vi "DCP SORT.vi"(11 "Clusters in":T1) -> (3 "Array":string[][](array[string]))   [LabVIEW 2015]
uses:
  TypeDefs/DCP and LLDP Cluster.ctl
  TypeDefs/DCP ARRAY.ctl
  TypeDefs/Profinet Ident.ctl
  TypeDefs/LLDP ARRAY.ctl
  TypeDefs/LLDP.ctl
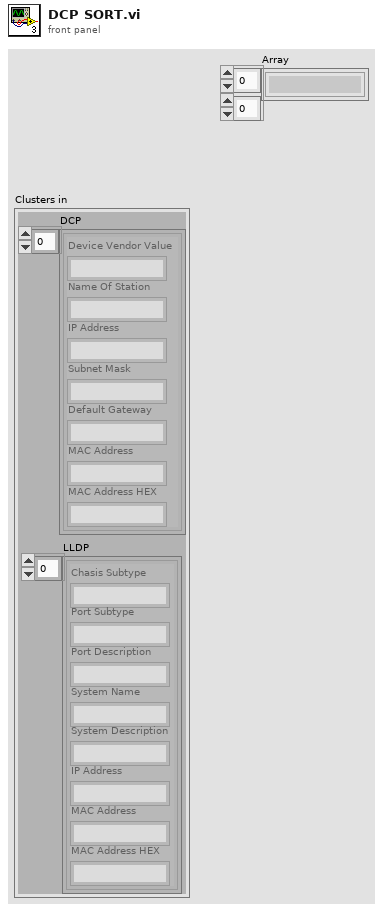
[diagram p1: front panel]
types:
  T1 = typedef "DCP and LLDP Cluster.ctl" = cluster{"DCP":T2, "LLDP":T4}
  T2 = typedef "DCP ARRAY.ctl" = T3[]
  T3 = typedef "Profinet Ident.ctl" = cluster{"Device Vendor Value":string, "Name Of Station":string, "IP Address":string, "Subnet Mask":string, "Default Gateway":string, "MAC Address":string, "MAC Address HEX":string}
  T4 = typedef "LLDP ARRAY.ctl" = T5[]
  T5 = typedef "LLDP.ctl" = cluster{"Chasis Subtype":string, "Port Subtype":string, "Port Description":string, "System Name":string, "System Description":string, "IP Address":string, "MAC Address":string, "MAC Address HEX":string}
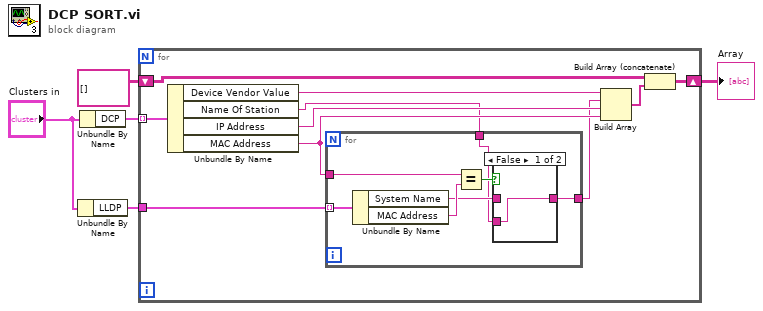
[diagram p0: block diagram]
diagram:
  n1 = Unbundle By Name("Clusters in") -> ("LLDP"=w2:T4)
  n2 = Unbundle By Name("Clusters in") -> ("DCP"=w4:T2)
  n3 = for {
    tunnel: w4 -> [w15] mode=indexing
    shift-right: [w12] -> w5
    shift-left: string[][] [] -> [w11]
    tunnel: w2 -> [w10]
    n4 = Unbundle By Name(w15) -> ("Device Vendor Value"=w8:string, "Name Of Station"=w7:string, "IP Address"=w14:string, "MAC Address"=w9:string)
    n5 = for {
      tunnel: w10 -> [w22] mode=indexing
      tunnel: w9 -> [w21]
      tunnel: [w17] -> w6
      tunnel: w7 -> [w16]
      n6 = Unbundle By Name(w22) -> ("System Name"=w18:string, "MAC Address"=w20:string)
      n7 = Equal?(x=w21, y=w20) -> (x = y?=w19:bool)
      n8 = case shown="False" w19 {
        tunnel: w18 -> [_ w24]
        tunnel: [w23 w24] -> w17
        tunnel: w16 -> [w23 _]
        frame False {
        }
        frame True {
        }
      }
    }
    n9 = Build Array(w8, w6, w14, w9) -> (w13:string[])
    n10 = Build Array (concatenate)(w11, w13) -> (w12:string[][])
  }
  "Array" <- w5
